vi "Explode.vi"(11 "Asteroid in":refnum<class "Asteroid.lvclass">) -> (3 "Asteroid out":refnum<class "Asteroid.lvclass">)   [LabVIEW 2021, in "Asteroid.lvclass"]
uses:
  Asteroid.lvclass
  Asteroid.lvclass/Asteroid.ctl
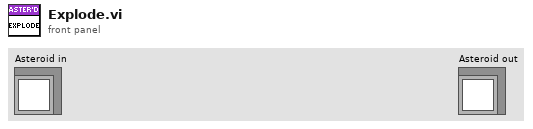
[diagram p1: front panel]
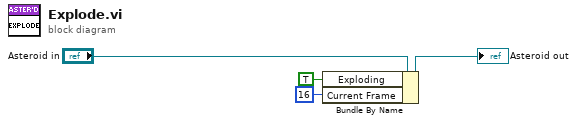
[diagram p0: block diagram]
diagram:
  n1 = Bundle By Name(cluster="Asteroid in", "Exploding"=TRUE, "Current Frame"=16) -> (→"Asteroid out":refnum<class "Asteroid.lvclass">)
